vi "rql_Whack Watchdog.vi"(4 "Show in Debugger?":bool=TRUE, 6 "Message Priority":T1=enum."Normal", 8 "error in":errorcluster, 10 "Data in":T2, 11 "RT Watchdog in":refnum<class "RT Watchdog.lvclass">) -> (0 "error out":errorcluster, 3 "dup RT Watchdog out":refnum<class "RT Watchdog.lvclass">)   [LabVIEW 2017, in "RT Watchdog.lvclass"]
doc: "This VI sends a <b>Local API Request</b> message to an MHL case of the Worker that owns this VI.\n---\nResets the watchdog counter to the value you specify using either the Watchdog Configure VI or the Watchdog Set Attribute VI."
uses:
  RT Watchdog.lvclass
  C:/Program Files (x86)/National Instruments/LabVIEW 2017/vi.lib/addons/_Workers/Library/Classes/Worker/Worker.lvclass
  rql_Whack Watchdog.ctl
  <vilib>/addons/_Workers/Library/Classes/Message/Priority.ctl
  <vilib>/addons/_Workers/Library/Case Label.ctl
  <vilib>/addons/_Workers/Library/Classes/Message Queue/Message Queue.lvclass
  <vilib>/addons/_Workers/Library/Workers.lvlib
  <vilib>/addons/_Workers/Library/Classes/Message/Message.lvclass
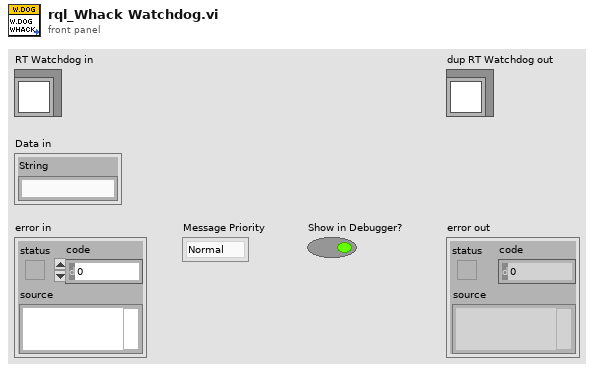
[diagram p1: front panel]
types:
  T1 = typedef "Workers.lvlib/Message.lvclass/Priority.ctl" = enum16{"Low", "Normal", "High"}
  T2 = typedef "RT Watchdog.lvclass/rql_Whack Watchdog.ctl" = cluster{"String":string}
  T3 = typedef "Workers.lvlib/Case Label.ctl" = string
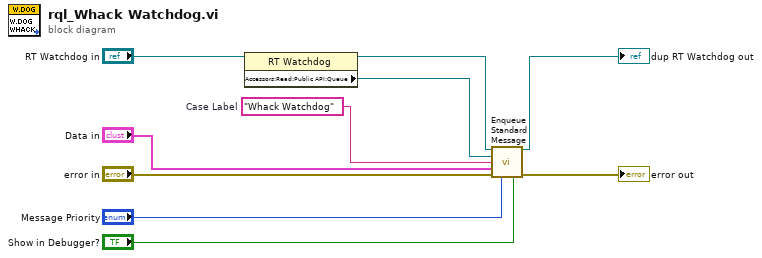
[diagram p0: block diagram]
diagram:
  w1 = T3 "Whack Watchdog"  # Case Label
  n1 = property class="RT Watchdog"(reference="RT Watchdog in") -> (reference out=w3:refnum<class "RT Watchdog.lvclass">, "Accessors:Read:Public API:Queue"=w2:refnum<class "Message Queue.lvclass">)  [unwired: 1 in, 1 out]
  n2 = call-dynamic "Enqueue Standard Message.vi"("Worker"=w3, "Message Queue"=w2, "Case Label"=w1, "Data"="Data in", "error in (no error)"="error in", "Priority (Normal)"="Message Priority", "Send Message to Debugger? (T)"="Show in Debugger?") -> ("dup Worker out"=→"dup RT Watchdog out":refnum<class "RT Watchdog.lvclass">, "error out"=→"error out":errorcluster)  [unwired: 7 in]
